vi "PutArray.vi"(8 "error in (no error)":errorcluster, 10 "Array":variant, 11 "MsgPackSerializer in":refnum<class "MsgPackSerializer.lvclass">) -> (0 "error out":errorcluster, 3 "MsgPackSerializer out":refnum<class "MsgPackSerializer.lvclass">)   [LabVIEW 2015, in "MsgPackSerializer.lvclass"]
uses:
  MsgPackSerializer.lvclass
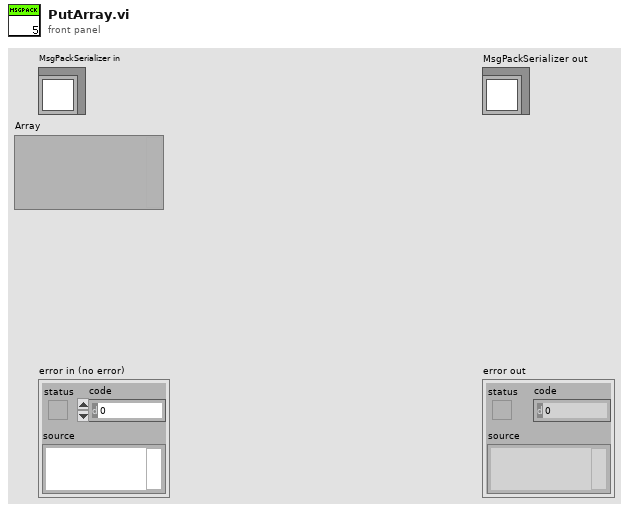
[diagram p1: front panel]
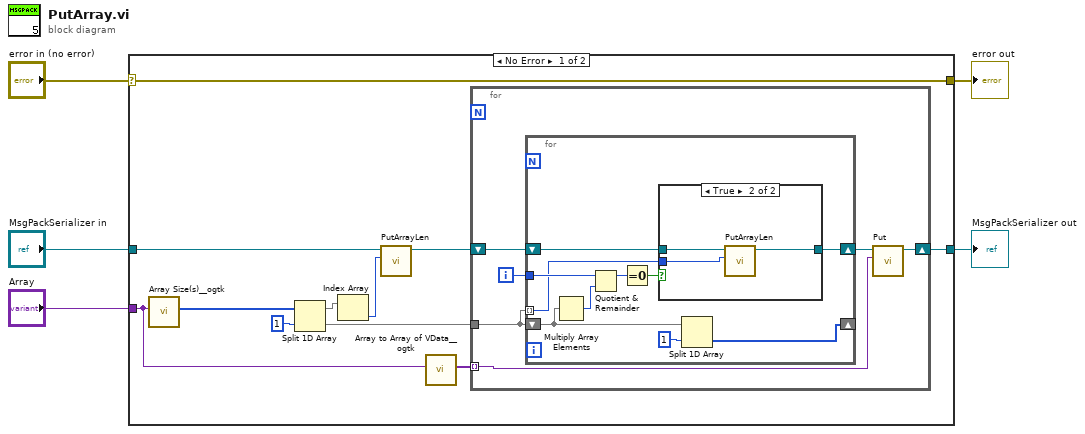
[diagram p0: block diagram]
diagram:
  n1 = case shown="No Error" "error in (no error)" {
    selector: "error in (no error)" -> [w16 w38]
    tunnel: [w16 w38] -> w4
    tunnel: [w15 w37] -> w2
    tunnel: "MsgPackSerializer in" -> [w14 w37]
    tunnel: "Array" -> [w12 _]
    frame No Error {
      n2 = call <userlib>:"Array Size(s)__ogtk.vi"("Array"=w12) -> ("Size(s)"=w9:u32[])  [unwired: 8 in, 2 out]
      n3 = Split 1D Array(array=w9, index=1) -> (first subarray=w7:u32[], second subarray=w8:u32[])
      n4 = Index Array(array=w7) -> (element=w6:u32)  [unwired: 1 in]
      n5 = call "PutArrayLen.vi"("len"=w6, "MsgPackSerializer in"=w14) -> ("MsgPackSerializer out"=w13:refnum<class "MsgPackSerializer.lvclass">)  [unwired: 8 in, 1 out]
      n6 = call <userlib>:"Array to Array of VData__ogtk.vi"("MultiD Array"=w12) -> ("1D Array of Variants"=w11:variant[])  [unwired: 9 in, 1 out]
      n7 = for {
        tunnel: w11 -> [w22] mode=indexing
        shift-right: [w17] -> w15
        shift-left: w13 -> [w19]
        tunnel: w8 -> [w20]
        i -> [w21]
        n8 = for {
          tunnel: w20 -> [w25] mode=indexing
          tunnel: w21 -> [w31]
          shift-right: [w27] -> _
          shift-left: w20 -> [w26]
          shift-right: [w23] -> w18
          shift-left: w19 -> [w24]
          n9 = Multiply Array Elements(1:w26) -> (0:w30:u32)
          n10 = Quotient & Remainder(x=w31, y=w30) -> (x-y*floor(x/y)=w29:u32)  [unwired: 1 out]
          n11 = Equal To 0?(x=w29) -> (x = 0?=w28:bool)
          n12 = case shown="True" w28 {
            tunnel: w25 -> [_ w36]
            tunnel: w24 -> [w33 w35]
            tunnel: [w33 w34] -> w23
            frame False {
            }
            frame True {
              n13 = call "PutArrayLen.vi"("len"=w36, "MsgPackSerializer in"=w35) -> ("MsgPackSerializer out"=w34:refnum<class "MsgPackSerializer.lvclass">)  [unwired: 8 in, 1 out]
            }
          }
          n14 = Split 1D Array(array=w26, index=1) -> (second subarray=w27:u32[])  [unwired: 1 out]
        }
        n15 = call "Put.vi"("Data"=w22, "MsgPackSerializer in"=w18) -> ("MsgPackSerializer out"=w17:refnum<class "MsgPackSerializer.lvclass">)  [unwired: 8 in, 1 out]
      }
    }
    frame Error {
    }
  }
  "error out" <- w4
  "MsgPackSerializer out" <- w2
